vi "Read Camera Temperature.vi"(8 "error in (no error)":errorcluster, 11 "Hamamatsu_C9100-13 in":refnum<class "Hamamatsu_C9100-13.lvclass">) -> (0 "error out":errorcluster, 2 "Camera Temperature":dbl, 3 "Hamamatsu_C9100-13 out":refnum<class "Hamamatsu_C9100-13.lvclass">)   [LabVIEW 2013, in "Hamamatsu_C9100-13.lvclass"]
uses:
  Hamamatsu_C9100-13.lvclass
  Hamamatsu_C9100-13.lvclass/Hamamatsu_C9100-13.ctl
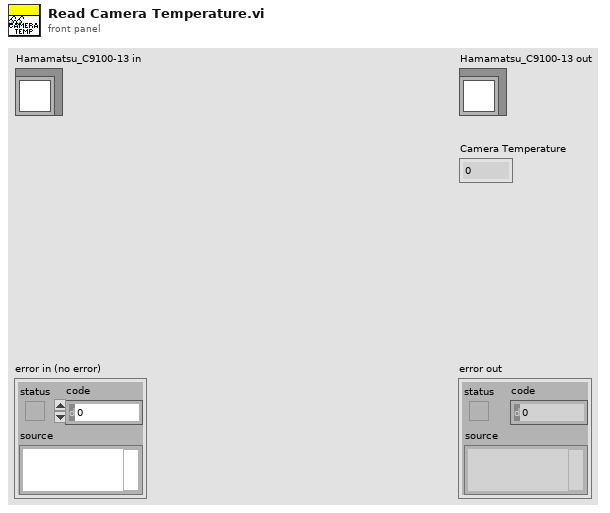
[diagram p1: front panel]
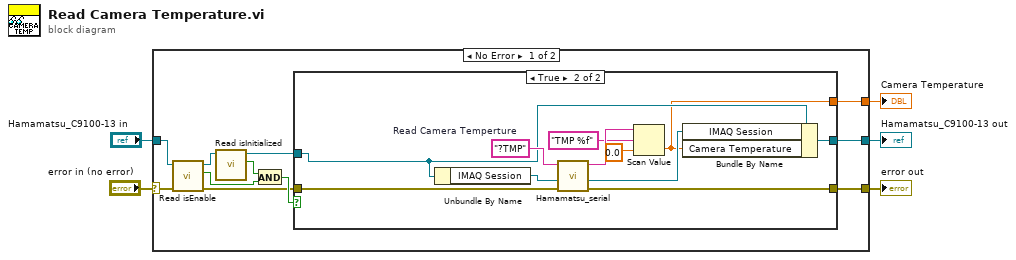
[diagram p0: block diagram]
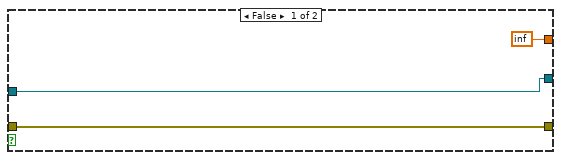
[diagram p2: hidden frame]
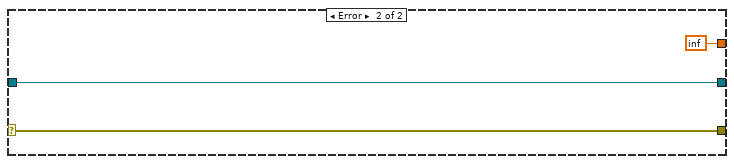
[diagram p3: hidden frame]
diagram:
  n1 = case shown="No Error" "error in (no error)" {
    selector: "error in (no error)" -> [w8 w32]
    tunnel: [w16 w32] -> w4
    tunnel: "Hamamatsu_C9100-13 in" -> [w10 w33]
    tunnel: [w14 inf] -> w2
    tunnel: [w15 w33] -> w1
    frame No Error {
      n2 = call-dynamic "Read isEnable.vi"("error in (no error)"=w8, "Camera in"=w10) -> ("error out"=w7:errorcluster, "Use camera?"=w6:bool, "Camera out"=w9:refnum<class "Hamamatsu_C9100-13.lvclass">)  [unwired: 7 in]
      n3 = call-dynamic "Read isInitialized.vi"("Camera in"=w9) -> ("isInitialized?"=w11:bool, "Camera out"=w13:refnum<class "Hamamatsu_C9100-13.lvclass">)  [unwired: 8 in, 1 out]
      n4 = And(x=w11, y=w6) -> (x .and. y?=w12:bool)
      n5 = case shown="True" w12 {
        tunnel: w7 -> [w19 w27]
        tunnel: [w19 w26] -> w16
        tunnel: [w18 w24] -> w15
        tunnel: [inf w20] -> w14
        tunnel: w13 -> [w18 w21]
        frame False {
        }
        frame True {
          w28 = "?TMP"  # Read Camera Temperture
          n6 = Unbundle By Name(w21) -> ("IMAQ Session"=w25:refnum<k11>)
          n7 = call "Hamamatsu_serial.vi"("error in"=w27, "IMAQ Session In"=w25, "Command to send"=w28) -> ("error out"=w26:errorcluster, "IMAQ Session Out"=w23:refnum<k11>, "Response from Camera"=w30:string)  [unwired: 6 in]
          n8 = Scan Value(string=w30, format string="TMP %f", default (0 dbl)=0.0 ("value (0)")) -> (value=w20:dbl)  [unwired: 1 out]
          n9 = Bundle By Name(cluster=w21, "IMAQ Session"=w23, "Camera Temperature"=w20) -> (w24:refnum<class "Hamamatsu_C9100-13.lvclass">)
        }
      }
    }
    frame Error {
    }
  }
  "error out" <- w4
  "Hamamatsu_C9100-13 out" <- w1
  "Camera Temperature" <- w2
